vi "Get Obj Data.vi"(0 "reference in":refnum<class "Nastran PCH.lvclass">, 5 "error in (no error)":errorcluster) -> (13 "FRF":T1(array[cluster]), 14 "reference out":refnum<class "Nastran PCH.lvclass">, 19 "error out":errorcluster)   [LabVIEW 2022 SP3, in "Nastran PCH.lvclass"]
uses:
  Nastran PCH.lvclass
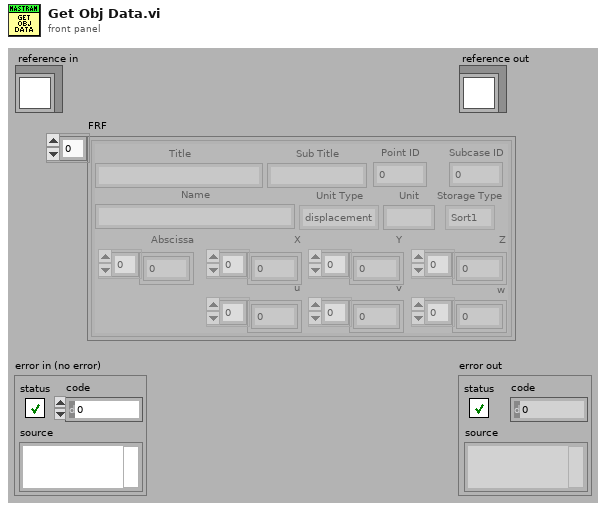
[diagram p1: front panel]
types:
  T1 = cluster{"Title":string, "Sub Title":string, "Point ID":i32, "Subcase ID":i32, "Name":string, "Unit Type":enum16{"displacement", "velocity", "acceleration"}, "Unit":string, "Storage Type":enum16{"Sort1", "Sort2"}, "Abscissa":dbl[], "X":cdb[], "Y":cdb[], "Z":cdb[], "u":cdb[], "v":cdb[], "w":cdb[]}[]
  T2 = typedef "Nastran PCH.lvclass/ObjectAttributes.ctl" = cluster{"FRF":cluster{"Title":string, "Sub Title":string, "Point ID":i32, "Subcase ID":i32, "Name":string, "Unit Type":enum16{"displacement", "velocity", "acceleration"}, "Unit":string, "Storage Type":enum16{"Sort1", "Sort2"}, "Abscissa":dbl[], "X":cdb[], "Y":cdb[], "Z":cdb[], "u":cdb[], "v":cdb[], "w":cdb[]}[]}
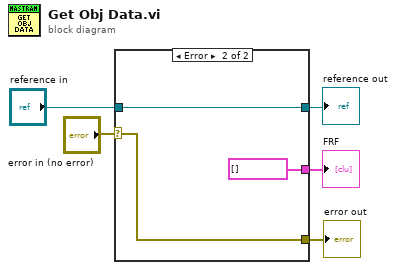
[diagram p0: block diagram]
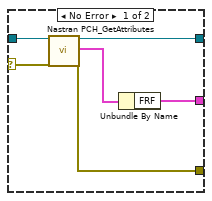
[diagram p2: hidden frame]
diagram:
  n1 = case shown="Error" "error in (no error)" {
    selector: "error in (no error)" -> [w11 w14]
    tunnel: [w10 w14] -> w4
    tunnel: [w9 w13] -> w2
    tunnel: "reference in" -> [w7 w13]
    tunnel: [w6 T1 [] ("FRF")] -> w1
    frame No Error {
      n2 = call "Nastran PCH_GetAttributes.vi"("reference in"=w7, "error in (no error)"=w11) -> ("reference out"=w9:refnum<class "Nastran PCH.lvclass">, "attributes"=w8:T2, "error out"=w10:errorcluster)  [unwired: 14 in, 1 out]
      n3 = Unbundle By Name(w8) -> ("FRF"=w6:T1)
    }
    frame Error {
    }
  }
  "error out" <- w4
  "reference out" <- w2
  "FRF" <- w1
